vi "TSE_Callback.vi"(4 "User Parameter":variant, 5 "Event Data":cluster{"uiMsg":refnum<k7>}, 6 "Control Ref":refnum<k7>, 7 "Event Common Data":T1) -> ()   [LabVIEW 2014]
uses:
  VeriPaylasim_Globali.vi
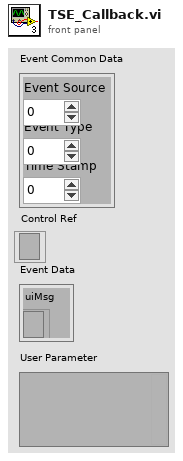
[diagram p1: front panel]
types:
  T1 = cluster{"Event Source":i32, "Event Type":u32, "Time Stamp":u32}
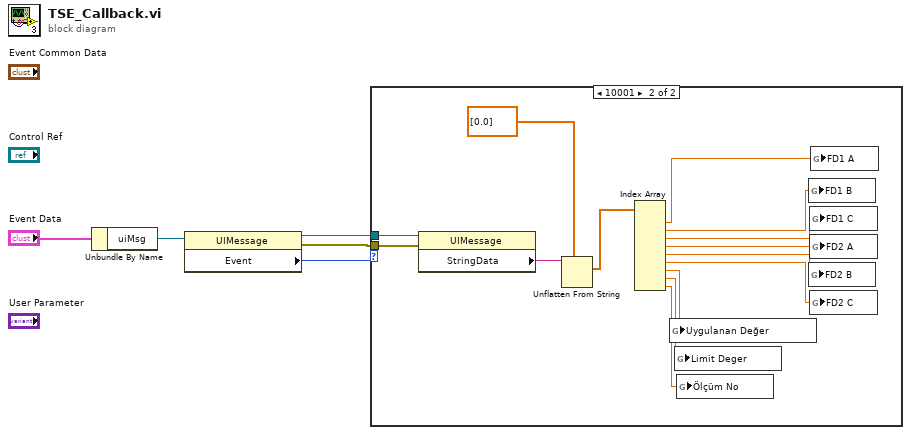
[diagram p0: block diagram]
diagram:
  n1 = Unbundle By Name("Event Data") -> ("uiMsg"=w4:refnum<k7>)
  n2 = property class="UIMessage"(reference=w4) -> (reference out=w2:refnum<k7>, error out=w1:errorcluster, "Event"=w3:i32)  [unwired: 1 in]
  n3 = case shown="10001" w3 {
    tunnel: w2 -> [_ w19]
    tunnel: w1 -> [_ w18]
    frame 0, Default {
    }
    frame 10001 {
      n4 = property class="UIMessage"(reference=w19, error in=w18) -> ("StringData"=w8:string)  [unwired: 2 out]
      n5 = Unflatten From String(type=dbl[] [0.0], binary string=w8) -> (value=w6:dbl[])  [unwired: 3 in, 2 out]
      n6 = Index Array(array=w6) -> (element #1=w17:dbl, element #2=w16:dbl, element #3=w15:dbl, element #4=w14:dbl, element #5=w13:dbl, element #6=w12:dbl, element #7=w11:dbl, element #8=w10:dbl, element #9=w9:dbl)  [unwired: 9 in]
      n7 = global write "VeriPaylasim_Globali.vi" "Uygulanan Değer"(w11) -> ()
      n8 = global write "VeriPaylasim_Globali.vi" "Limit Deger"(w10) -> ()
      n9 = global write "VeriPaylasim_Globali.vi" "Ölçüm No"(w9) -> ()
      n10 = global write "VeriPaylasim_Globali.vi" "FD1 B"(w16) -> ()
      n11 = global write "VeriPaylasim_Globali.vi" "FD2 B"(w13) -> ()
      n12 = global write "VeriPaylasim_Globali.vi" "FD1 C"(w15) -> ()
      n13 = global write "VeriPaylasim_Globali.vi" "FD2 A"(w14) -> ()
      n14 = global write "VeriPaylasim_Globali.vi" "FD2 C"(w12) -> ()
      n15 = global write "VeriPaylasim_Globali.vi" "FD1 A"(w17) -> ()
    }
  }
